vi "oopAPI_TX (UDP Port-Oriented)_2.vi"() -> ()   [LabVIEW 2020]
uses:
  src/_polimorphicInstances/control/Fdx Start (Tx).vi
  src/AIM664LV.lvlib
  src/_polimorphicInstances/session/Fdx Close Session (Port).vi
  src/_polimorphicInstances/session/Fdx Create Session (Tx-UDP Port-Oriented).vi
  src/bsp/AFDX_Transmit/Fdx Create Tx VL.vi
  src/_polimorphicInstances/udpPort/Fdx Create UDP Port (TX-CommPort).vi
  src/_polimorphicInstances/control/Fdx Stop (Tx).vi
  src/_controls/comm_computedMAC-IP.ctl
  src/_controls/comm_udp_tx.ctl
  src/_controls/comm_config_vl_tx.ctl
panel:
  out "Duplicated":bool
  in  "VL Config":T1={"VlId"=60, "NumOfSubVl"=2, "rate mS (128)"=128.0, "domainID"=1, "sideID"=1, "locationID"=1, "interfaceID"=1, "NetSelect"=3, "Skew"=0, "MaxFrameLength"=1000, "FrameBufferSize"=0} {"NetSelect" items=["FDX_TX_FRAME_DLY_A"=0, "FDX_TX_FRAME_DLY_B"=1, "FDX_TX_FRAME_BOTH "=3, "FDX_TX_FRAME_ONLY_A"=4, "FDX_TX_FRAME_ONLY_B "=5]; "interfaceID" format="%.0b"}
  in  "CommPort Config":T2[](array[typedef])=[{"PortType"=enum."FDX_UDP_SAMPLING", "partitionID"=1, "SubVlId"=1, "UdpSrcPort"=1, "UdpDstPort"=1, "SampleRateMs"=128.0, "UdpNumBufMessages"=0, "UdpMaxMessageSize"=1000}, {"PortType"=enum."FDX_UDP_SAMPLING", "partitionID"=1, "SubVlId"=2, "UdpSrcPort"=2, "UdpDstPort"=2, "SampleRateMs"=128.0, "UdpNumBufMessages"=0, "UdpMaxMessageSize"=1000}]
  in  "millisecond multiple":u32=128
  in  "PortMap":u32
  out "IndexCycleCount":u32[](array[numeric])
  out "MsgCount":u32[](array[numeric])
  out "CurrentIndex":u32[](array[numeric])
  out "BytesWritten":u32[](array[numeric])
  in  "port":u32
  in  "board":u32
  out "current time":timestamp=timestamp(3677762637.591913 s since 1904-01-01)
  out "current irig time":T3={"SignOut"=40, "DayOut"=1, "HourOut"=1, "MinOut"=28, "SecondOut"=39, "MilliSecOut"=539, "MicroSecOut"=300, "NanoSecOut"=0, "InfoOut"=0, "Mode"=3}
  out "CommPort Addresses":T4[](array[typedef]) {"MACsrc" format="%.0x"}
  in  "Data":u8[](array[numeric])=[255, 255, 255, 255, 255, 255, 255, 255, 255, 255, 255, 255, 255, 255, 255, 255, 255, 255, 255, 255, 255, 255, 255, 255, 255, 255, 255, 255, 255, 255, 255, 255, 255, 255, 255, 255, 255, 255, 255, 255, 255, 255, 255, 255, 255, 255, 255, 255, 255, 255, 255, 255, 255, 255, 255, 255, 255, 255, 255, 255, 255, 255, 255, 255, 255, 255, 255, 255, 255, 255, 255, 255, 255, 255, 255, 255, 255, 255, 255, 255, 255, 255, 255, 255, 255, 255, 255, 255, 255, 255, 255, 255, 255, 255, 255, 255, 255, 255, 255, 170] format="%.0x"
  in  "stop":bool
  out "PortInitOut":T5={"PortConfig"=0, "PortUsed"=1, "GlobalMemFree"=0, "SharedMemFree"=0} {"PortConfig" items=["FDX_SINGLE", "FDX_REDUNDANT"]}
  out "error out":errorcluster
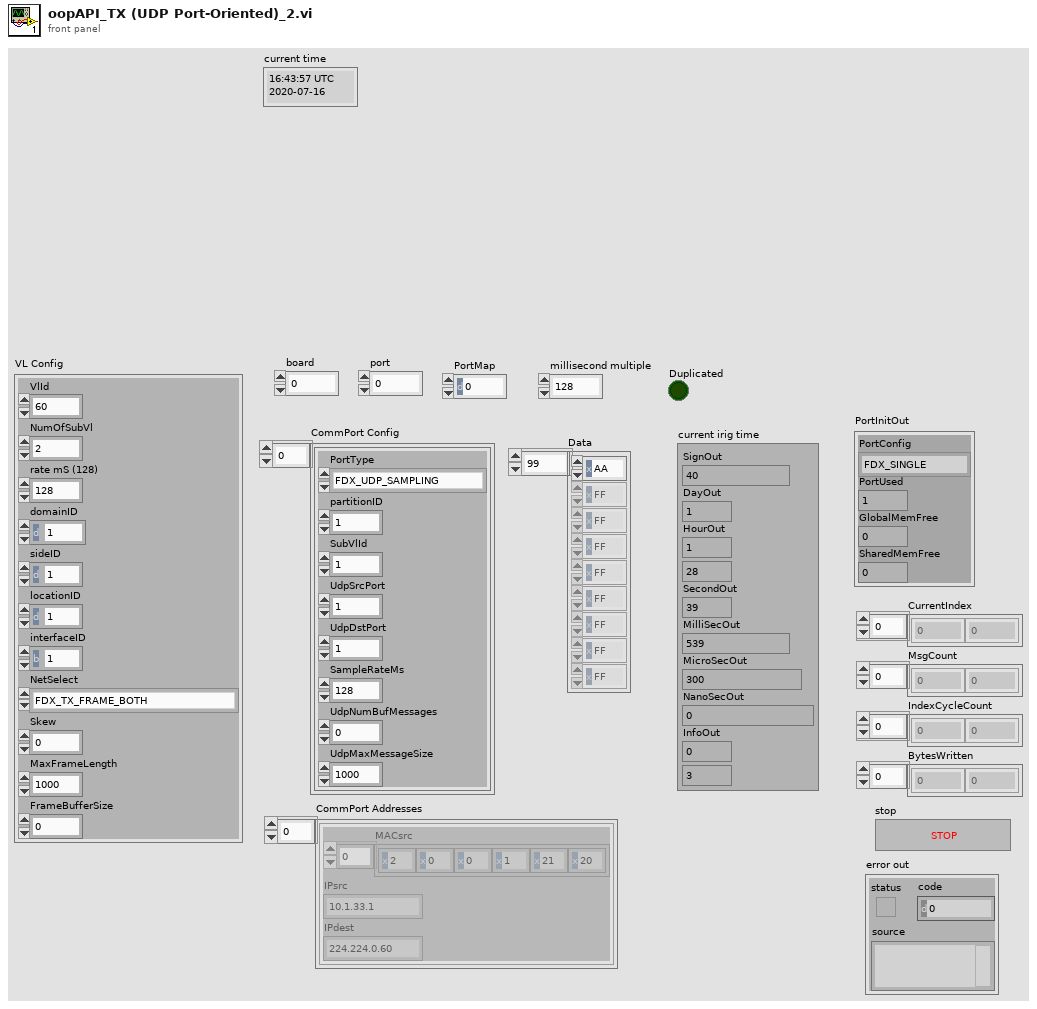
[diagram p1: front panel]
types:
  T1 = typedef "AIM664LV.lvlib/comm_config_vl_tx.ctl" = cluster{"VlId":u16, "NumOfSubVl":u16, "rate mS (128)":dbl, "domainID":u8, "sideID":u8, "locationID":u8, "interfaceID":u8, "NetSelect":u32, "Skew":u32, "MaxFrameLength":u32, "FrameBufferSize":u32}
  T2 = typedef "AIM664LV.lvlib/comm_udp_tx.ctl" = cluster{"PortType":enum16{"FDX_UDP_SAMPLING", "FDX_UDP_QUEUING"}, "partitionID":u8, "SubVlId":u8, "UdpSrcPort":u16, "UdpDstPort":u16, "SampleRateMs":dbl, "UdpNumBufMessages":u32, "UdpMaxMessageSize":u32}
  T3 = cluster{"SignOut":i32, "DayOut":u32, "HourOut":u32, "MinOut":u32, "SecondOut":u32, "MilliSecOut":u32, "MicroSecOut":u32, "NanoSecOut":u32, "InfoOut":u32, "Mode":u32}
  T4 = typedef "AIM664LV.lvlib/comm_computedMAC-IP.ctl" = cluster{"MACsrc":u8[], "IPsrc":string, "IPdest":string}
  T5 = cluster{"PortConfig":u32, "PortUsed":u32, "GlobalMemFree":u32, "SharedMemFree":u32}
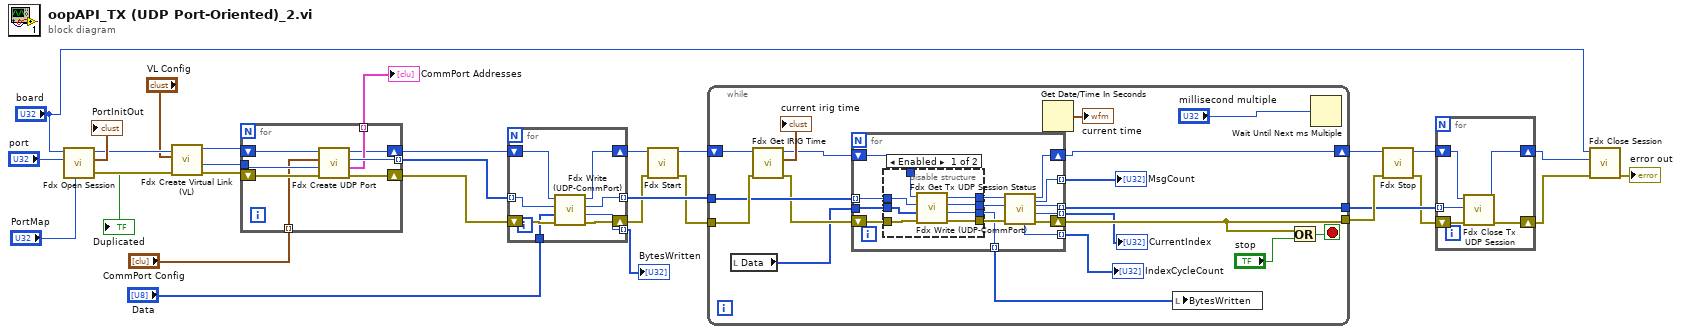
[diagram p0: block diagram]
diagram:
  n1 = call-poly "Fdx Open Session.vi"("PortMap"="PortMap", "port"="port", "board"="board") -> ("error out"=w12:errorcluster, "PortInitOut"=→"PortInitOut":T5, "port handle out"=w13:u32, "Duplicated"=→"Duplicated":bool)  [unwired: 4 in, 1 out]
  n2 = call-poly "Fdx Create Virtual Link (VL).vi"("error in (no error)"=w12, "VL Config"="VL Config", "InstrumentHandle in"=w13) -> ("error out"=w10:errorcluster, "VlId"=w9:u16, "InstrumentHandle out"=w11:u32)  [unwired: 6 in]
  n3 = for {
    tunnel: [w38] -> w29 mode=indexing
    tunnel: [w35] -> w25 mode=indexing
    shift-right: [w34] -> w4
    shift-left: w11 -> [w39]
    shift-right: [w37] -> w27
    shift-left: w10 -> [w36]
    tunnel: w9 -> [w33]
    tunnel: "CommPort Config" -> [w32] mode=indexing
    n4 = call-poly "Fdx Create UDP Port.vi"("error in (no error)"=w36, "VlId"=w33, "CommPort Config"=w32, "port handle in"=w39) -> ("error out"=w37:errorcluster, "computedAddresses"=w35:T4, "commPort handle out"=w38:u32, "port handle out"=w34:u32)  [unwired: 4 in]
  }
  "CommPort Addresses" <- w25
  n5 = for {
    tunnel: "Data" -> [w43]
    tunnel: [w45] -> w15 mode=indexing
    shift-right: [w46] -> w23
    shift-left: w27 -> [w47]
    tunnel: w29 -> [w44] mode=indexing
    tunnel: [w40] -> w28 mode=indexing
    shift-right: [w41] -> w3
    shift-left: w4 -> [w42]
    n6 = call "Fdx Write (UDP-CommPort).vi"("error in (no error)"=w47, "Data"=w43, "UdpHandle in"=w44, "InstrumentHandle_port in"=w42) -> ("error out"=w46:errorcluster, "BytesWritten"=w45:u32, "UdpHandle out"=w40:u32, "InstrumentHandle_port out"=w41:u32)  [unwired: 4 in]
  }
  "BytesWritten" <- w15
  n7 = call-poly "Fdx Start.vi"("error in (no error)"=w23, "InstrumentHandle_port in"=w3) -> ("error out"=w22:errorcluster, "InstrumentHandle_port out"=w21:u32)  [unwired: 8 in]
  n8 = while {
    tunnel: w22 -> [w61]
    tunnel: w28 -> [w53]
    tunnel: [w58] -> w18
    tunnel: [w57] -> w19
    shift-right: [w48] -> w24
    shift-left: w21 -> [w62]
    stop <- w64 stop-if-true
    n9 = local read "Data"() -> (w50:u8[])
    n10 = call "Fdx Get IRIG Time.vi"("error in (no error)"=w61, "InstrumentHandle_board in"=w62) -> ("error out"=w52:errorcluster, "Curent Irig Time"=→"current irig time":T3, "InstrumentHandle_board out"=w49:u32)  [unwired: 7 in]
    n11 = for {
      tunnel: [w67] -> w58 mode=indexing
      tunnel: [w78] -> w56 mode=indexing
      tunnel: [w68] -> w55 mode=indexing
      tunnel: [w77] -> w54 mode=indexing
      tunnel: w53 -> [w76] mode=indexing
      tunnel: [w72] -> w51 mode=indexing
      tunnel: w50 -> [w71]
      shift-right: [w79] -> w57
      shift-left: w52 -> [w75]
      shift-right: [w66] -> w48
      shift-left: w49 -> [w70]
      n12 = disable-structure shown="Enabled" {
        disable-tunnel: w76 -> [w81 w89]
        disable-tunnel: w75 -> [w87 w88]
        disable-tunnel: [w86 w88] -> w74
        disable-tunnel: [w82 w89] -> w73
        disable-tunnel: [w85 _] -> w72
        disable-tunnel: w71 -> [w80 _]
        disable-tunnel: w70 -> [w84 _]
        disable-tunnel: [w83 _] -> w69
        frame Enabled {
          n13 = call "Fdx Write (UDP-CommPort).vi"("error in (no error)"=w87, "Data"=w80, "UdpHandle in"=w81, "InstrumentHandle_port in"=w84) -> ("error out"=w86:errorcluster, "BytesWritten"=w85:u32, "UdpHandle out"=w83:u32, "InstrumentHandle_port out"=w82:u32)  [unwired: 4 in]
        }
        frame Disabled {
        }
      }
      n14 = call "Fdx Get Tx UDP Session Status.vi"("error in (no error)"=w74, "UdpHandle in"=w69, "InstrumentHandle_port in"=w73) -> ("error out"=w79:errorcluster, "CurrentIndex"=w78:u32, "UdpHandle out"=w67:u32, "InstrumentHandle_port out"=w66:u32, "IndexCycleCount"=w77:u32, "MsgCount"=w68:u32)  [unwired: 3 in]
    }
    "CurrentIndex" <- w56
    "MsgCount" <- w55
    "IndexCycleCount" <- w54
    n15 = Get Date/Time In Seconds() -> (seconds since 1Jan1904=→"current time":timestamp)
    n16 = local write "BytesWritten"(w51) -> ()
    n17 = Or(x=w57, y="stop") -> (x .or. y?=w64:bool)
    n18 = Wait Until Next ms Multiple(millisecond multiple="millisecond multiple") -> ()  [unwired: 1 out]
  }
  n19 = call-poly "Fdx Stop.vi"("error in (no error)"=w19, "InstrumentHandle_port in"=w24) -> ("error out"=w17:errorcluster, "InstrumentHandle_port out"=w2:u32)  [unwired: 8 in]
  n20 = for {
    tunnel: w18 -> [w92] mode=indexing
    shift-right: [w93] -> w16
    shift-left: w17 -> [w94]
    shift-right: [w90] -> w1
    shift-left: w2 -> [w91]
    n21 = call "Fdx Close Tx UDP Session.vi"("error in (no error)"=w94, "UdpHandle in"=w92, "InstrumentHandle_port in"=w91) -> ("error out"=w93:errorcluster, "InstrumentHandle_port out"=w90:u32)  [unwired: 7 in]
  }
  n22 = call-poly "Fdx Close Session.vi"("error in (no error)"=w16, "InstrumentHandle_port in"=w1, "InstrumentHandle_board in"="board") -> ("error out"=→"error out":errorcluster)  [unwired: 8 in]
